vi "HSFL1dll.vi"(8 "error in (no error)":errorcluster, 11 "Inputs":T2) -> (0 "error out":errorcluster, 3 "Outputs":T1)   [LabVIEW 2021]
uses:
  REFPROP.dll
panel:
  # "REFPROP-HSFL1dll.vi"
  # "void  HSFL1dll(double *h, double *s, double *z, double *dmin, double dmax, double t, double d, int32_t *ierr, CStr herr, int32_t herr_length);"
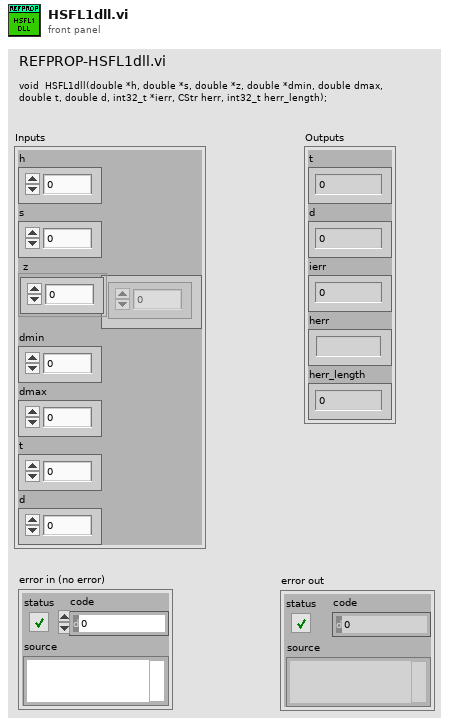
[diagram p1: front panel]
types:
  T1 = cluster{"t ":dbl, "d":dbl, "ierr":i32, "herr":string, "herr_length":i32}
  T2 = cluster{"h":dbl, "s":dbl, "z":dbl[], "dmin":dbl, "dmax":dbl, "t":dbl, "d":dbl}
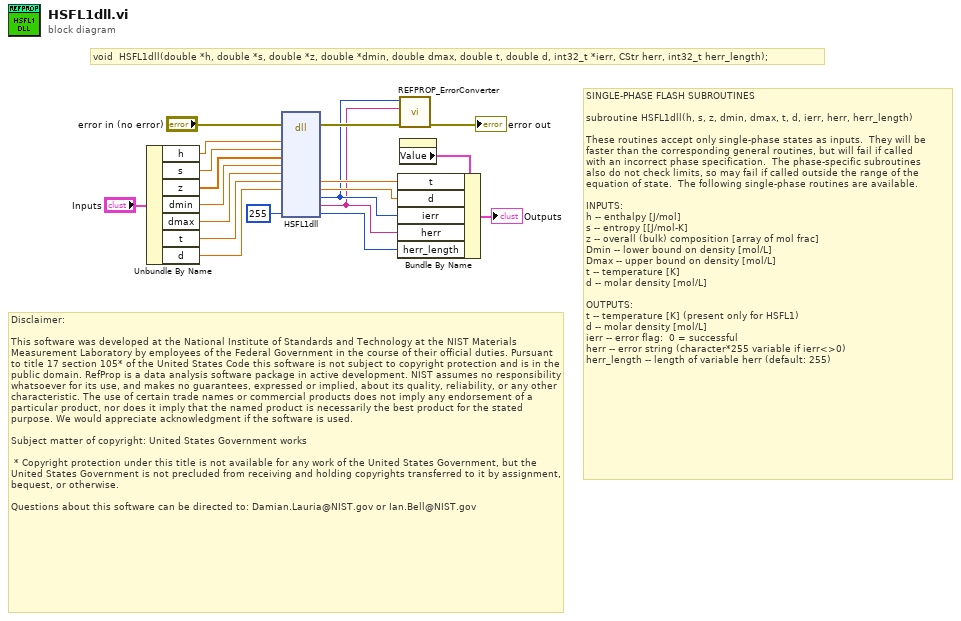
[diagram p0: block diagram]
diagram:
  # "Disclaimer:\n\nThis software was developed at the National Institute of Standards and Technology at the NIST Materials Measurement Laboratory by employees of the Federal Government in the course of their official duties. Pursuant to title 17 section 105* of the United States Code this software is not subject to copyright protection and is in the public domain. RefProp is a data analysis software package in active development. NIST assumes no responsibility whatsoever for its use, and makes no guarantees, expressed or implied, about its quality, reliability, or any other characteristic. The use of certain trade names or commercial products does not imply any endorsement of a particular product, nor does it imply that the named product is necessarily the best product for the stated purpose. We would appreciate acknowledgment if the software is used.\n \nSubject matter of copyright: United States Government works\n  \n * Copyright protection under this title is not available for any work of the United States Government, but the United States Government is not precluded from receiving and holding copyrights transferred to it by assignment, bequest, or otherwise.\n\nQuestions about this software can be directed to: Damian.Lauria@NIST.gov or Ian.Bell@NIST.gov"
  # "void  HSFL1dll(double *h, double *s, double *z, double *dmin, double dmax, double t, double d, int32_t *ierr, CStr herr, int32_t herr_length);"
  # "SINGLE-PHASE FLASH SUBROUTINES\n\nsubroutine HSFL1dll(h, s, z, dmin, dmax, t, d, ierr, herr, herr_length) \n\nThese routines accept only single-phase states as inputs.  They will be\nfaster than the corresponding general routines, but will fail if called\nwith an incorrect phase specification.  The phase-specific subroutines\nalso do not check limits, so may fail if called outside the range of the\nequation of state.  The following single-phase routines are available.\n\nINPUTS: \nh -- enthalpy [J/mol]\ns -- entropy [[J/mol-K]\nz -- overall (bulk) composition [array of mol frac]\nDmin -- lower bound on density [mol/L]\nDmax -- upper bound on density [mol/L]\nt -- temperature [K]\nd -- molar density [mol/L]\n\nOUTPUTS:\nt -- temperature [K] (present only for HSFL1)\nd -- molar density [mol/L]\nierr -- error flag:  0 = successful\nherr -- error string (character*255 variable if ierr<>0)\nherr_length -- length of variable herr (default: 255)"
  n1 = Unbundle By Name("Inputs") -> ("h"=w14:dbl, "s"=w13:dbl, "z"=w12:dbl[], "dmin"=w11:dbl, "dmax"=w10:dbl, "t"=w9:dbl, "d"=w8:dbl)
  n2 = dll-call lib="C:/Users/lauria/OneDrive - National Institute of Standards and Technology (NIST)/LabVIEW Projects/7 REFPROP/REFPROP-wrappers-master/REFPROP-wrappers-master/wrappers/Labview/REFPROP/REFPROP.*" fn="HSFL1dll"(error in="error in (no error)", "h"=w14, "s"=w13, "z"=w12, "dmin"=w11, "dmax"=w10, "t"=w9, "d"=w8, "herr_length"=255) -> (error out=w18:errorcluster, "t"=w5:dbl, "d"=w4:dbl, "ierr"=w3:i32, "herr"=w2:string, "herr_length"=w1:i32)  [unwired: 10 in, 1 out]
  n3 = call "REFPROP_ErrorConverter.vi"("error in (no error)"=w18, "Error Message"=w2, "Error Code"=w3) -> ("error out"=→"error out":errorcluster)  [unwired: 8 in]
  n4 = property on="Outputs" class="Clust (strict)"() -> ("Value"=w7:T1)  [unwired: 2 in, 2 out]
  n5 = Bundle By Name(cluster=w7, "t"=w5, "d"=w4, "ierr"=w3, "herr"=w2, "herr_length"=w1) -> (→"Outputs":T1)
